vi "SeCrTs-RD Log Digital Queues.vi"(8 "error in":errorcluster, 9 "DI_queue":refnum<queue>[](array[refnum]), 10 "DI Names":string[](array[string]), 11 "tdms file in":refnum<k34>) -> (0 "error out":errorcluster, 3 "tdms file out":refnum<k34>)   [LabVIEW 2022 SP3]
uses:
  <vilib>/Waveform/DWDTOps.llb/DWDT Digital to Analog.vi
  <vilib>/Waveform/DWDTOps.llb/DWDT Get Waveform Time Array.vi
panel:
  out "max queue size":i32
  out "# elements in queue":i32
  out "# pending insert":i32
  out "# pending remove":i32
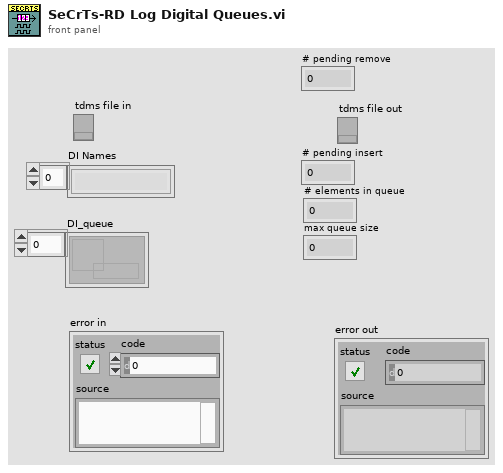
[diagram p1: front panel]
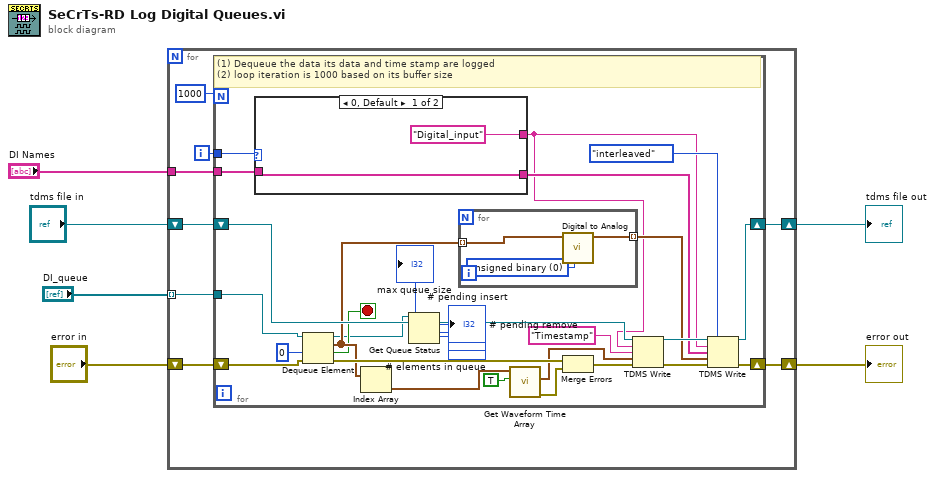
[diagram p0: block diagram]
diagram:
  n1 = for {
    tunnel: "DI_queue" -> [w11] mode=indexing
    tunnel: "DI Names" -> [w8]
    shift-right: [w9] -> w2
    shift-left: "error in" -> [w14]
    shift-right: [w10] -> w3
    shift-left: "tdms file in" -> [w13]
    i -> [w7]
    n2 = for {
      N: 1000 -> [_]
      shift-right: [w31] -> w10
      shift-left: w13 -> [w33]
      shift-right: [w36] -> w9
      shift-left: w14 -> [w39]
      tunnel: w11 -> [w24]
      tunnel: w8 -> [w23]
      tunnel: w7 -> [w22]
      stop <- w27 stop-if-true
      # "(1) Dequeue the data its data and time stamp are logged\n(2) loop iteration is 1000 based on its buffer size"
      n3 = case shown="0, Default" w22 {
        tunnel: w23 -> [w44 _]
        tunnel: [w44 _] -> w21
        tunnel: ["Digital_input" ("group name in (Untitled)") _] -> w20
        frame 0, Default {
        }
        frame 1 {
        }
      }
      n4 = Dequeue Element(queue=w24, timeout in ms (-1)=0, error in (no error)=w39) -> (queue out=w19:refnum<queue>, element=w29:digitalwaveform[], timed out?=w27:bool, error out=w41:errorcluster)
      n5 = Index Array(array=w29) -> (element=w25:digitalwaveform)  [unwired: 1 in]
      n6 = Get Queue Status(queue=w19) -> (max queue size=→"max queue size":i32, # pending remove=→"# pending remove":i32, # pending insert=→"# pending insert":i32, # elements in queue=→"# elements in queue":i32)  [unwired: 2 in, 4 out]
      n7 = for {
        tunnel: w29 -> [w47] mode=indexing
        tunnel: [w46] -> w28 mode=indexing
        w45 = u16 0 items=["unsigned binary", "offset binary", "2's complement"] ("data format (offset binary)")
        n8 = call-poly <vilib>:"Digital to Analog.vi"("data format (offset binary)"=w45, "digital waveform"=w47) -> ("analog waveform"=w46:waveform(dbl))  [unwired: 6 in, 3 out]
      }
      n9 = call-poly <vilib>:"Get Waveform Time Array.vi"("match transition array"=TRUE, "waveform in"=w25) -> ("error out"=w40:errorcluster, "X array"=w34:timestamp[])  [unwired: 8 in]
      n10 = Merge Errors(w41, w40) -> (w38:errorcluster)
      n11 = TDMS Write(0:w33, 5:w20, 7:"Timestamp", 9:w34, 11:w38) -> (4:w32:refnum<k34>, 15:w37:errorcluster)  [unwired: 1 in, 2 out]
      n12 = TDMS Write(0:w32, 1:enum16{"decimated", "interleaved"}."interleaved" ("data layout (0:decimated)"), 5:w20, 7:w21, 9:w28, 11:w37) -> (4:w31:refnum<k34>, 15:w36:errorcluster)  [unwired: 2 out]
    }
  }
  "tdms file out" <- w3
  "error out" <- w2
